vi "SvgDoc Open.vi"(8 "error in":errorcluster, 11 "SVG":path) -> (0 "error out":errorcluster, 3 "SVG out":refnum<k24>)   [LabVIEW 2020, in "SvgDotNet.lvlib"]
uses:
  SvgDotNet.lvlib
  C:/Users/huipeng8/Desktop/SVG.NET/Svg.dll
  Svg.dll
panel:
  # "Connector Pane"
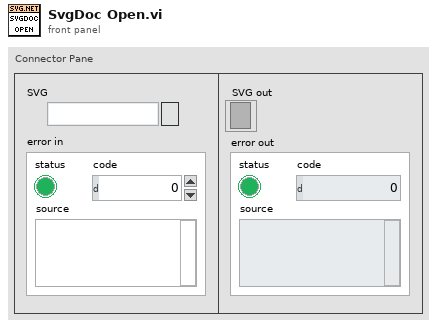
[diagram p1: front panel]
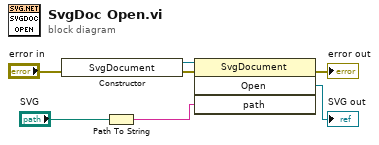
[diagram p0: block diagram]
diagram:
  n1 = constructor class="SvgDocument"(error in="error in") -> (reference out=w4:refnum<k24>, error out=w5:errorcluster)  [unwired: 2 in, 1 out]
  n2 = Path To String(path="SVG") -> (string=w3:string)
  n3 = invoke class="SvgDocument" method="Open"(reference=w4, error in=w5, "path"=w3) -> (error out=→"error out":errorcluster, "Open"=→"SVG out":refnum<k24>)  [unwired: 1 in, 2 out]
